vi "Is Flat Type.vi"(8 "error in (no error)":errorcluster, 11 "LVAnalogWaveformType in":refnum<class "LVAnalogWaveformType.lvclass">) -> (0 "error out":errorcluster, 2 "Flat Type?":bool, 3 "LVAnalogWaveformType out":refnum<class "LVAnalogWaveformType.lvclass">)   [LabVIEW 2020, in "LVDataTypes.lvlib" / "LVAnalogWaveformType.lvclass"]
uses:
  <vilib>/AppBuilder/Engine/WebServiceDescription/LVDataTypes/LVAnalogWaveformType/LVAnalogWaveformType.lvclass
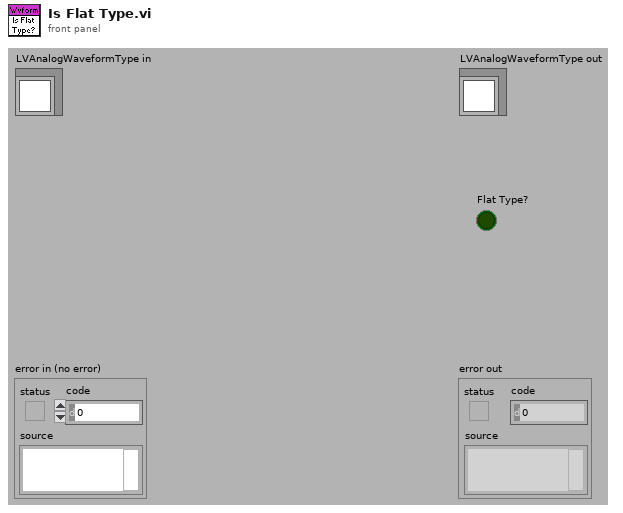
[diagram p1: front panel]
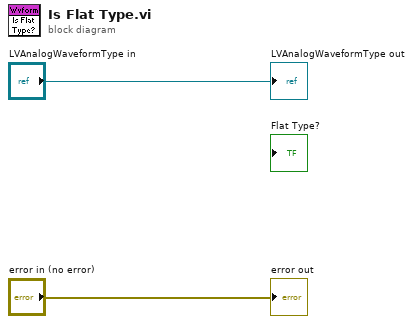
[diagram p0: block diagram]
diagram:
  "error out" <- "error in (no error)"
  "LVAnalogWaveformType out" <- "LVAnalogWaveformType in"
